vi "Array Mania.vi"() -> ()   [LabVIEW 2017]
uses:
  <vilib>/Analysis/Matrix/Datatypes/RealMatrix.ctl
  83ae2fe0-6230-43da-bdbf-e8aff4b9e75e.vi
  32947982-e3a5-4f78-bc2d-f3ddbf658eec.vi
  d41ce4d9-4482-4c04-9365-0dd0685b8d49.vi
  <vilib>/Analysis/Matrix/Numeric/Conversions/Matrix To Array - RM.vi
  <vilib>/Analysis/Matrix/NI_Matrix.lvlib
panel:
  out "Real 2D Array":dbl[][](array[numeric])
  out "appended array":T1
  out "array (last n elements first)":string[](array[string])
  out "y value":dbl
  out "array out 2":dbl[](array[numeric])
  out "array out":dbl[](array[numeric])
  out "interleaved array":string[](array[string])
  out "decimated array 3":string[](array[string])
  out "decimated array 2":string[](array[string])
  out "decimated array":string[](array[string])
  out "second subarray":string[](array[string])
  out "first subarray":string[](array[string])
  out "reversed array":string[](array[string])
  out "shuffled array":string[](array[string])
  out "index of element":i32
  out "sorted array 2":string[](array[string])
  in  "Array":string[](array[string])
  out "sorted array":dbl[](array[numeric])
  out "output array":dbl[](array[numeric])
  out "min index(es)":i32
  out "min value":dbl
  out "max index(es)":i32
  out "max value":dbl
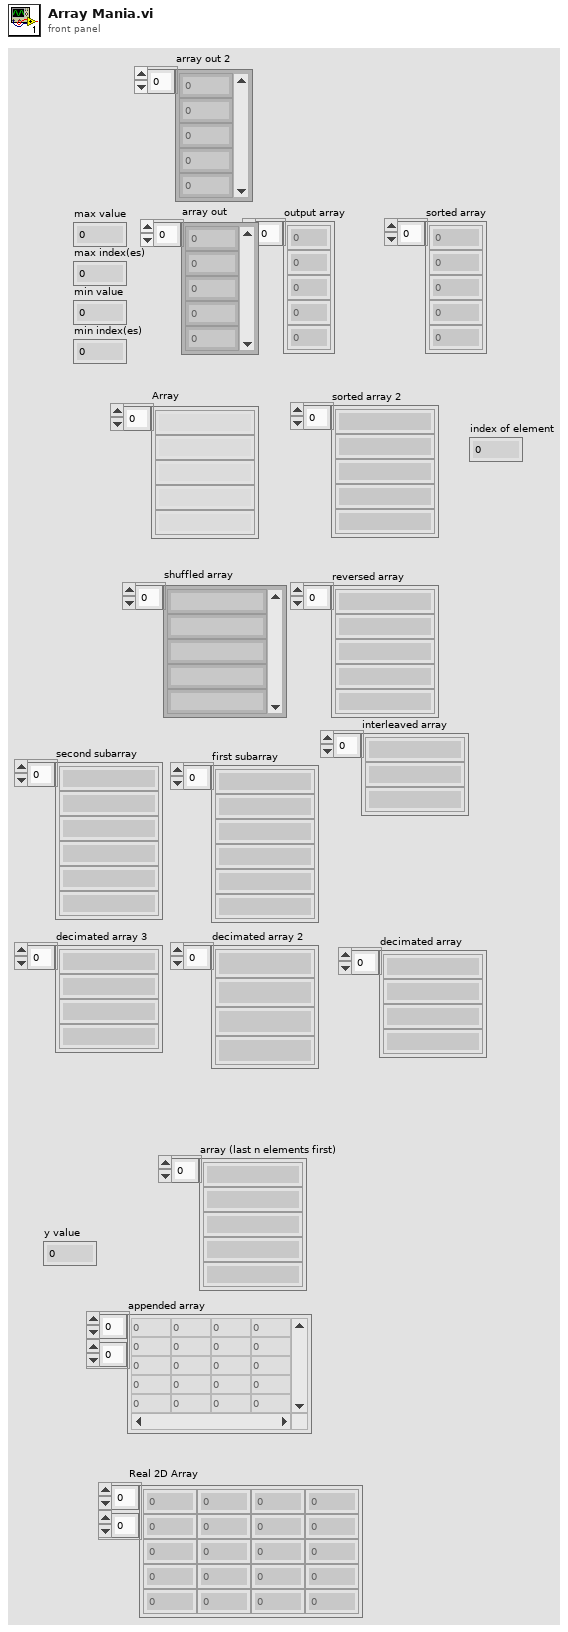
[diagram p1: front panel]
types:
  T1 = typedef "NI_Matrix.lvlib/RealMatrix.ctl" = dbl[][]
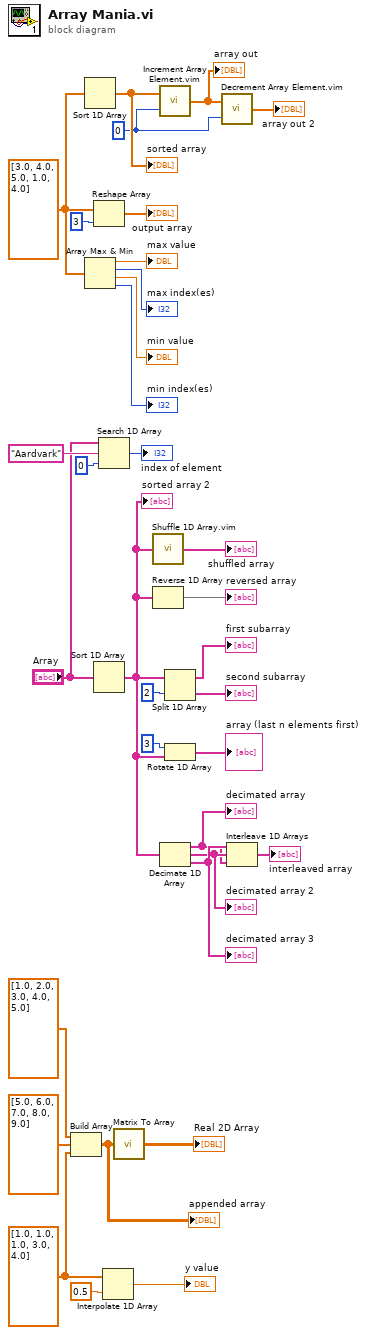
[diagram p0: block diagram]
diagram:
  w3 = dbl[] [1.0, 1.0, 1.0, 3.0, 4.0] ("array of numbers or points")
  w14 = 0 ("index")
  w12 = dbl[] [3.0, 4.0, 5.0, 1.0, 4.0] ("array")
  n1 = Build Array(dbl[] [1.0, 2.0, 3.0, 4.0, 5.0] ("element"), dbl[] [5.0, 6.0, 7.0, 8.0, 9.0] ("element"), w3) -> (w2:T1)
  "appended array" <- w2
  n2 = Sort 1D Array(array=w12) -> (sorted array=w16:dbl[])
  "sorted array" <- w16
  n3 = Array Max & Min(array=w12) -> (max value=→"max value":dbl, max index (indices)=→"max index(es)":i32, min value=→"min value":dbl, min index (indices)=→"min index(es)":i32)
  n4 = Reshape Array(w12, 3 ("dimension size")) -> (→"output array":dbl[])
  n5 = Sort 1D Array(array="Array") -> (sorted array=w6:string[])
  "sorted array 2" <- w6
  n6 = Search 1D Array(1D array="Array", element="Aardvark", start index (0)=0) -> (index of element=→"index of element":i32)
  n7 = Interpolate 1D Array(1:0.5 ("fractional index or x"), 2:w3) -> (0:→"y value":dbl)
  n8 = call-poly <vilib>:"Matrix To Array.vi"("Real Matrix"=w2) -> ("Real 2D Array"=→"Real 2D Array":dbl[][])
  n9 = call "Shuffle 1D Array.vim"("array"=w6) -> ("shuffled array"=→"shuffled array":string[])  [unwired: 4 in]
  n10 = Reverse 1D Array(array=w6) -> (reversed array=→"reversed array":string[])
  n11 = call "Increment Array Element.vim"("index"=w14, "array in"=w16) -> ("array out"=w15:dbl[])
  "array out" <- w15
  n12 = Decimate 1D Array(w6) -> (w18:string[], w19:string[], w20:string[])
  "decimated array" <- w18
  "decimated array 2" <- w19
  "decimated array 3" <- w20
  n13 = Split 1D Array(array=w6, index=2) -> (first subarray=→"first subarray":string[], second subarray=→"second subarray":string[])
  n14 = Rotate 1D Array(1:w6, 2:3 ("n")) -> (0:→"array (last n elements first)":string[])
  n15 = call "Decrement Array Element.vim"("index"=w14, "array in"=w15) -> ("array out"=→"array out 2":dbl[])
  n16 = Interleave 1D Arrays(w20, w19, w18) -> (→"interleaved array":string[])
